vi "Slack-Receive OAuth Code.vi"(11 "error in (no error)":errorcluster) -> (4 "code":string, 15 "error out":errorcluster)   [LabVIEW 2020]
uses:
  <vilib>/regexp/Match Regular Expression.xnode
panel:
  out "Header":string
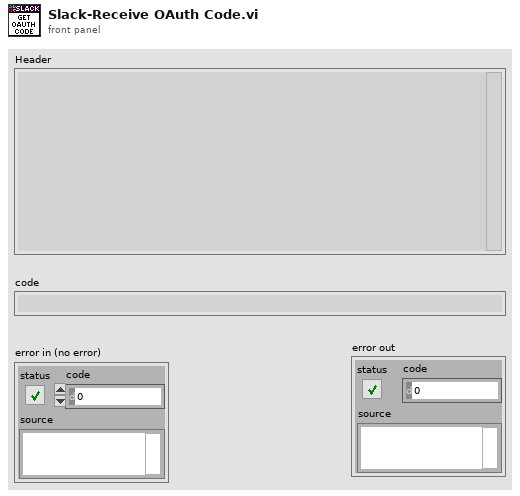
[diagram p1: front panel]
types:
  T1 = enum16{"Standard", "Buffered", "CRLF", "Immediate"}
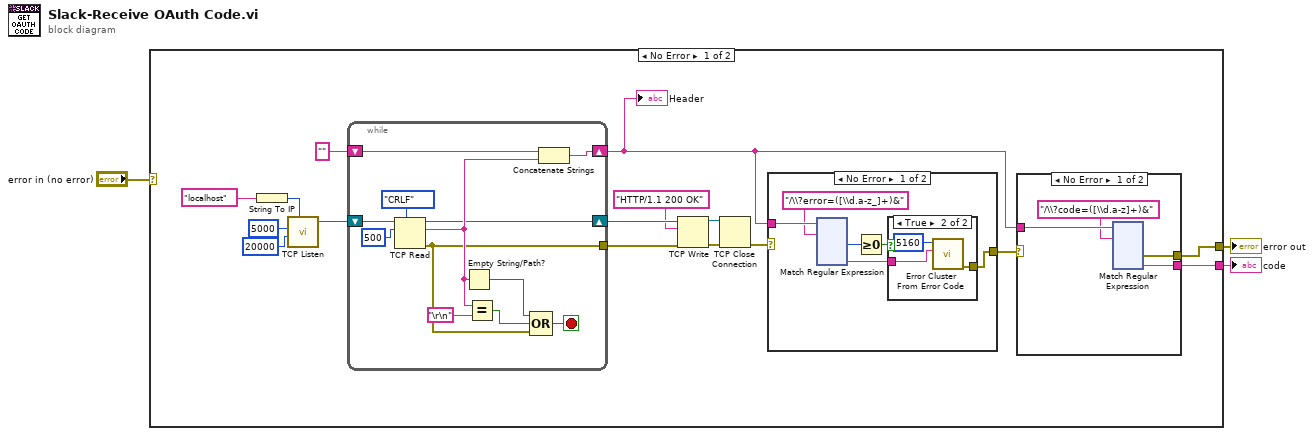
[diagram p0: block diagram]
diagram:
  n1 = case shown="No Error" "error in (no error)" {
    selector: "error in (no error)" -> [_ w279]
    tunnel: [w10 w279] -> w3
    tunnel: [w9 _] -> w2
    frame No Error {
      n2 = String To IP(1:"localhost") -> (0:w4:u32)
      n3 = call <vilib>:"TCP Listen.vi"("net address"=w4, "timeout ms (wait forever: -1)"=20000, "port"=u16 5000) -> ("connection ID"=w18:refnum<k5>)  [unwired: 4 in, 4 out]
      n4 = while {
        shift-right: [w274] -> w7
        shift-left: "" -> [w275]
        shift-right: [w268] -> w15
        shift-left: w18 -> [w278]
        tunnel: [w267] -> w11
        stop <- w269 stop-if-true
        n5 = TCP Read(connection ID=w278, bytes to read=500, 7:T1."CRLF" ("mode (standard)")) -> (connection ID out=w268:refnum<k5>, data out=w270:string, error out=w267:errorcluster)  [unwired: 2 in]
        n6 = Empty String/Path?(string/path=w270) -> (empty?=w271:bool)
        n7 = Equal?(x=w270, y="\r\n") -> (x = y?=w272:bool)
        n8 = Compound Arithmetic op=OR(w271, w272, w267) -> (w269:bool)
        n9 = Concatenate Strings(w275, w270) -> (w274:string)
      }
      "Header" <- w7
      n10 = TCP Write(connection ID=w15, data in="HTTP/1.1 200 OK", error in (no error)=w11) -> (connection ID out=w13:refnum<k5>, error out=w14:errorcluster)  [unwired: 1 in, 1 out]
      n11 = TCP Close Connection(connection ID=w13, error in (no error)=w14) -> (error out=w8:errorcluster)  [unwired: 1 in, 1 out]
      n12 = case shown="No Error" w8 {
        selector: w8 -> [_ w145]
        tunnel: w7 -> [w25 _]
        tunnel: [w20 w145] -> w6
        frame No Error {
          n13 = xnode "Match Regular Expression"("input string"=w25, "regular expression"="/\\?error=([\\d.a-z_]+)&") -> ("offset past match"=w21:i32, "submatch 1"=w23:string)  [unwired: 4 in, 4 out]
          n14 = Greater Or Equal To 0?(x=w21) -> (x >= 0?=w22:bool)
          n15 = case shown="True" w22 {
            tunnel: w23 -> [_ w27]
            tunnel: [_ w28] -> w20
            frame False {
            }
            frame True {
              n16 = call <vilib>:"Error Cluster From Error Code.vi"("error message (\"\")"=w27, "error code (0)"=5160) -> ("error out"=w28:errorcluster)  [unwired: 7 in]
            }
          }
        }
        frame Error {
        }
      }
      n17 = case shown="No Error" w6 {
        selector: w6 -> [_ w266]
        tunnel: w7 -> [w149 _]
        tunnel: [w147 w266] -> w10
        tunnel: [w146 _] -> w9
        frame No Error {
          n18 = xnode "Match Regular Expression"("input string"=w149, "regular expression"="/\\?code=([\\d.a-z]+)&") -> ("error out"=w147:errorcluster, "submatch 1"=w146:string)  [unwired: 4 in, 4 out]
        }
        frame Error {
        }
      }
    }
    frame Error {
    }
  }
  "error out" <- w3
  "code" <- w2
